vi "New_File.vi"(8 "error in (no error)":errorcluster, 9 "Path":path, 10 "Buffer in":string[](array[string]), 11 "Sequence in":string[](array[string])) -> (0 "error out":errorcluster, 1 "Sequence Caption":string, 2 "Buffer out":string[](array[string]), 3 "Sequence_out":string[](array[string]))   [LabVIEW 2021]
uses:
  <vilib>/Utility/file.llb/Write To Spreadsheet File (string).vi
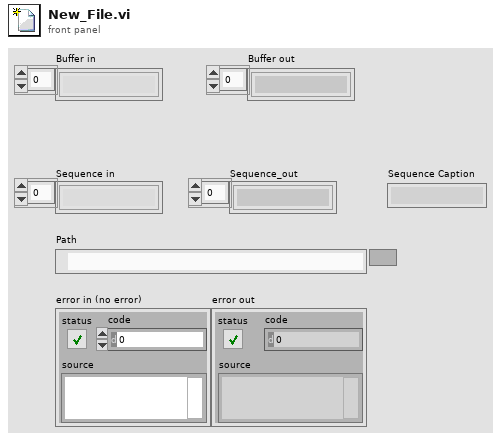
[diagram p1: front panel]
types:
  T1 = enum16{"Left Button", "Center Button", "Right Button", "Window Close"}
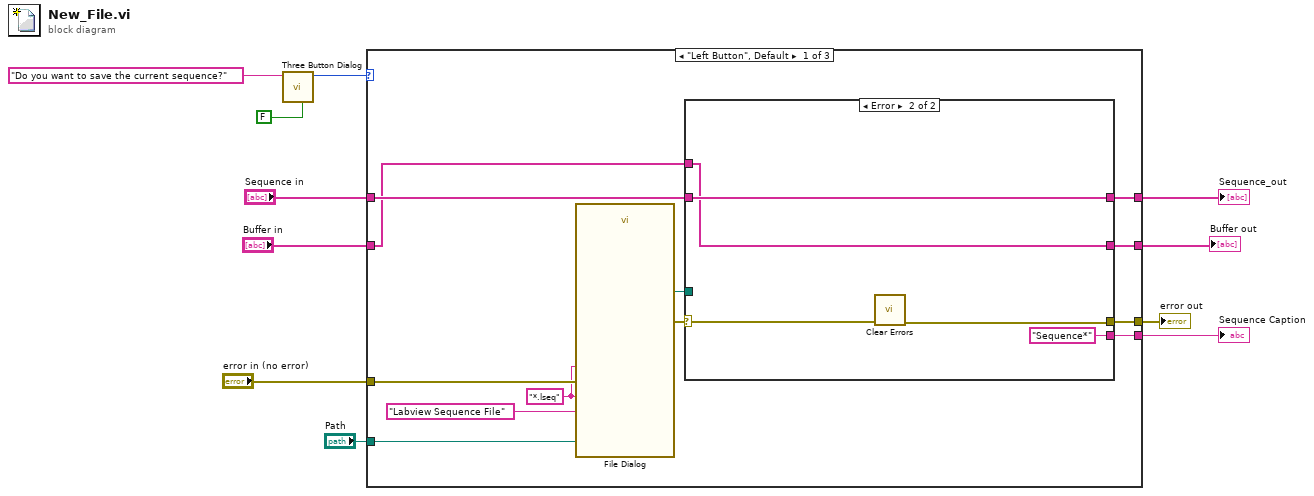
[diagram p0: block diagram]
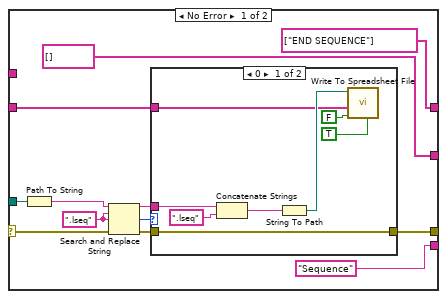
[diagram p2: hidden frame]
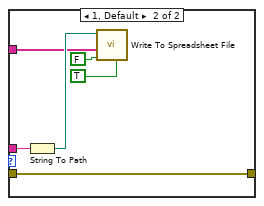
[diagram p3: hidden frame]
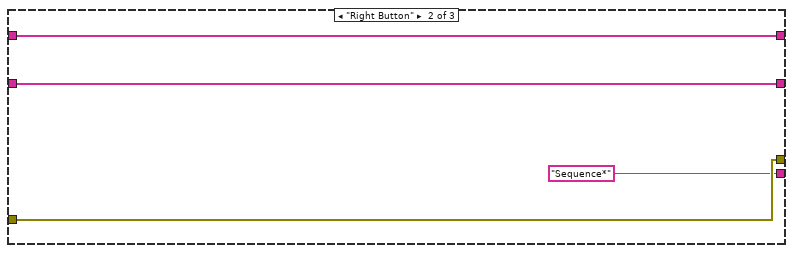
[diagram p4: hidden frame]
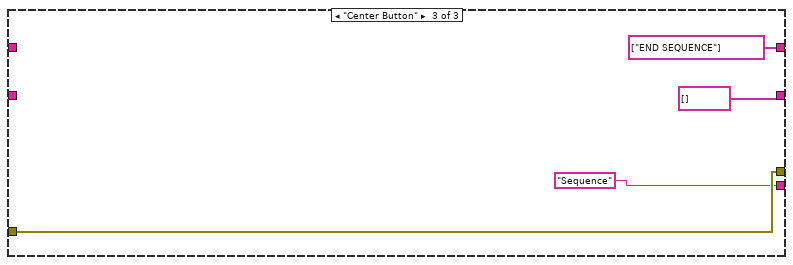
[diagram p5: hidden frame]
diagram:
  n1 = call <vilib>:"Three Button Dialog.vi"("Allow user to close window? (TRUE)"=FALSE, "message"="Do you want to save the current sequence?") -> ("Which Button?"=w9:T1)  [unwired: 9 in]
  n2 = case shown="\"Left Button\", Default" w9 {
    tunnel: "error in (no error)" -> [w22 w57 w62]
    tunnel: "Path" -> [w21 _ _]
    tunnel: [w19 w57 w62] -> w7
    tunnel: "Sequence in" -> [w17 w58 _]
    tunnel: [w15 w58 string[] ["END SEQUENCE"] ("Item Names")] -> w6
    tunnel: [w14 "Sequence*" "Sequence"] -> w3
    tunnel: "Buffer in" -> [w13 w55 _]
    tunnel: [w12 w55 string[] []] -> w1
    frame "Left Button", Default {
      w16 = "*.lseq"
      n3 = call "File Dialog"("start path"=w21, "default name"=w16, "error in"=w22, "pattern (all files)"=w16, "pattern label"="Labview Sequence File") -> ("selected path"=w18:path, "error out"=w20:errorcluster)  [unwired: 7 in, 2 out]
      n4 = case shown="Error" w20 {
        selector: w20 -> [w33 w51]
        tunnel: [w27 w50] -> w19
        tunnel: w18 -> [w35 _]
        tunnel: w17 -> [w29 w54]
        tunnel: [string[] ["END SEQUENCE"] ("Item Names") w54] -> w15
        tunnel: ["Sequence" "Sequence*"] -> w14
        tunnel: w13 -> [_ w52]
        tunnel: [string[] [] w52] -> w12
        frame No Error {
          w32 = ".lseq" ("search string")
          n5 = Path To String(path=w35) -> (string=w34:string)
          n6 = Search and Replace String(input string=w34, search string=w32, replace string=w32, error in=w33) -> (result string=w30:string, number of replacements=w31:i32, error out=w28:errorcluster)  [unwired: 4 in, 1 out]
          n7 = case shown="0" w31 {
            tunnel: w30 -> [w43 w44]
            tunnel: w29 -> [w39 w48]
            tunnel: w28 -> [w36 w45]
            tunnel: [w36 w45] -> w27
            frame 0 {
              n8 = Concatenate Strings(w43, ".lseq" ("string")) -> (w41:string)
              n9 = String To Path(string=w41) -> (path=w40:path)
              n10 = call-poly <vilib>:"Write To Spreadsheet File.vi"("transpose? (no:F)"=TRUE, "append to file? (new file:F)"=FALSE, "1D data"=w39, "file path (dialog if empty)"=w40) -> ()  [unwired: 4 in, 1 out]
            }
            frame 1, Default {
              n11 = String To Path(string=w44) -> (path=w49:path)
              n12 = call-poly <vilib>:"Write To Spreadsheet File.vi"("transpose? (no:F)"=TRUE, "append to file? (new file:F)"=FALSE, "1D data"=w48, "file path (dialog if empty)"=w49) -> ()  [unwired: 4 in, 1 out]
            }
          }
        }
        frame Error {
          n13 = call <vilib>:"Clear Errors.vi"("error in (no error)"=w51) -> ("error out"=w50:errorcluster)  [unwired: 5 in, 1 out]
        }
      }
    }
    frame "Right Button" {
    }
    frame "Center Button" {
    }
  }
  "error out" <- w7
  "Sequence_out" <- w6
  "Sequence Caption" <- w3
  "Buffer out" <- w1
